vi "GEA3 HEWH Full ERD List.vi"(0 "GEA2 Reference In":refnum<k24>, 11 "error in (no error)":errorcluster, 12 "Enable EMV List":bool, 13 "Enable Heat Pump List":bool, 14 "Enable Inverter ERD List":bool) -> (3 "GEA Inverter Inputs":T3 {"Destination" format="%.0x"; "Source" format="%.0x"}, 4 "GEA2 Reference Out":refnum<k24>, 6 "GEA MC Inputs":T3 {"Destination" format="%.0x"; "Source" format="%.0x"}, 8 "Read Inverter ERD List":T1[](array[typedef]) {"ERD Number" format="%.0x"}, 10 "Read MC ERD List":T1[](array[typedef]) {"ERD Number" format="%.0x"}, 15 "error out":errorcluster)   [LabVIEW 2020]
uses:
  type defs/ERD Read Data In.ctl
  type defs/Data Type.ctl
  type defs/Source_Destination.ctl
  C:/TechnologyLab/NI-2010/Drivers/GEA3 Toolkit/GEA3 DLL Source/GeaCommunication.dll
  GEA3 DLL Source/GeaCommunication.dll
  library/GEA2_Toolkit.lvlib
panel:
  out "Inverter Header":string[](array[string])
  out "MC Header":string[](array[string])
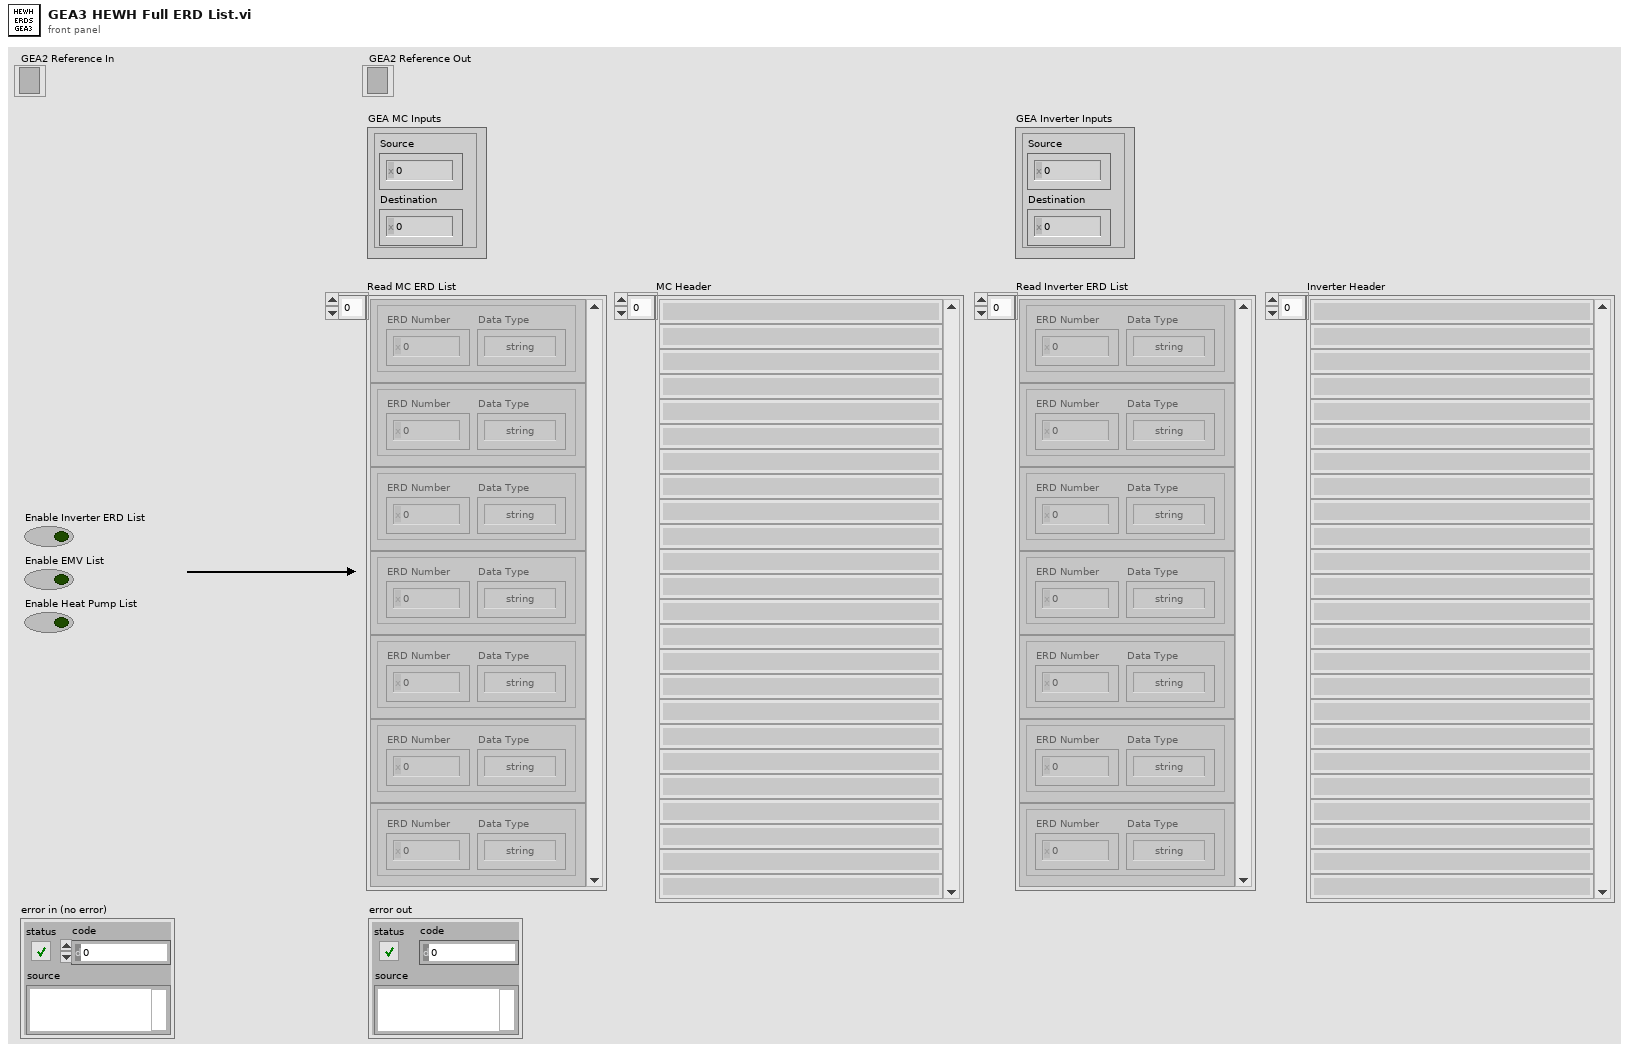
[diagram p1: front panel]
types:
  T1 = typedef "GEA2_Toolkit.lvlib/ERD Read Data In.ctl" = cluster{"ERD Number":u16, "Data Type":T2}
  T2 = typedef "GEA2_Toolkit.lvlib/Data Type.ctl" = enum16{"string", "boolean", "uint8_t", "uint16_t", "uint32_t", "uint64_t", "int8_t", "int16_t", "int32_t", "int64_t"}
  T3 = typedef "GEA2_Toolkit.lvlib/Source_Destination.ctl" = cluster{"Source":u8, "Destination":u8}
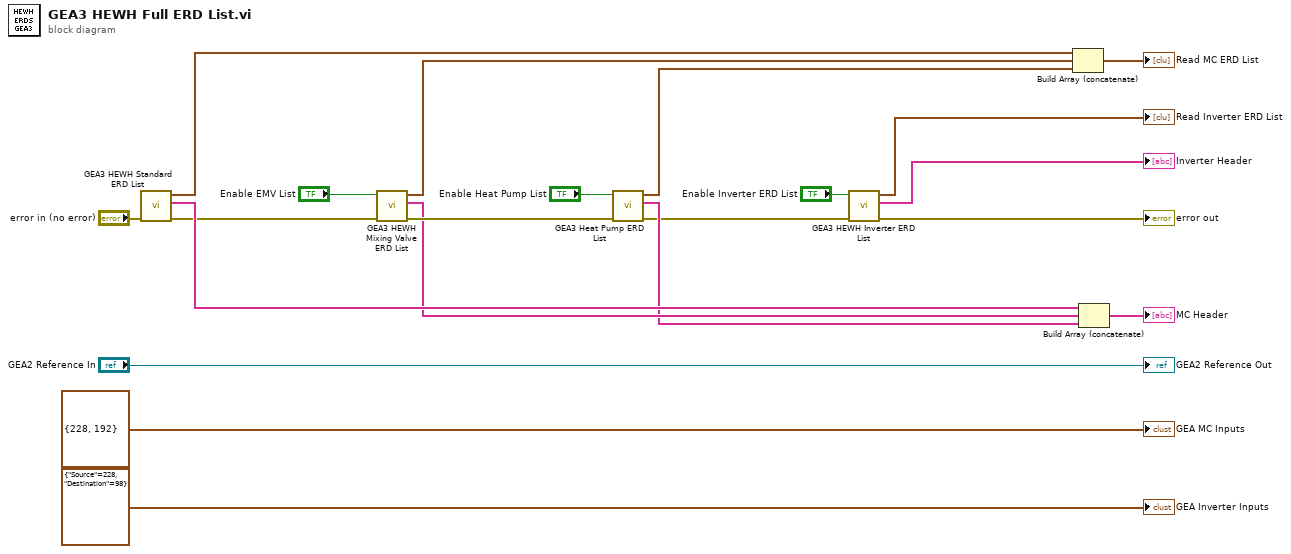
[diagram p0: block diagram]
diagram:
  n1 = call "GEA3 HEWH Standard ERD List.vi"("Error In"="error in (no error)") -> ("Error Out"=w3:errorcluster, "Header"=w11:string[], "Read ERD List"=w20:T1[])  [unwired: 8 in]
  n2 = call "GEA3 HEWH Mixing Valve ERD List.vi"("error in (no error)"=w3, "Enable Electronic Mixing Valve (EMV) List"="Enable EMV List") -> ("error out"=w14:errorcluster, "Headers"=w10:string[], "Read ERD List"=w18:T1[])  [unwired: 7 in]
  n3 = call "GEA3 Heat Pump ERD List.vi"("error in (no error)"=w14, "Enable Heat Pump List"="Enable Heat Pump List") -> ("error out"=w5:errorcluster, "Headers"=w9:string[], "Read ERD List"=w12:T1[])  [unwired: 7 in]
  n4 = call "GEA3 HEWH Inverter ERD List.vi"("error in (no error)"=w5, "Enable Inverter ERD List"="Enable Inverter ERD List") -> ("error out"=→"error out":errorcluster, "Headers"=→"Inverter Header":string[], "Read ERD List"=→"Read Inverter ERD List":T1[])  [unwired: 7 in]
  n5 = Build Array (concatenate)(w20, w18, w12) -> (→"Read MC ERD List":T1[])
  n6 = Build Array (concatenate)(w11, w10, w9) -> (→"MC Header":string[])
  "GEA MC Inputs" <- T3 {"Source"=228, "Destination"=192} ("GEA Inputs")
  "GEA2 Reference Out" <- "GEA2 Reference In"
  "GEA Inverter Inputs" <- T3 {"Source"=228, "Destination"=98} ("GEA Inputs")
